vi "LDA_High_Convert_New.vi"(1 "Analysis Info cluster":T2[](array[typedef]) {"Sync Delay Time (s)" format="%.4f"; "Total Meas Time (s)" format="%_5g"; "Sd Error in Variance" format="%_3g"; "Skew_u" format="%_3g"; "% u'/U" format="%_3g"; "Sd Error in Mean" format="%_3g"; "Kurt_u" format="%_3g"; "u^4" format="%_3g"; "u^3" format="%_3g"; "U" format="%_3g"; "u^2" format="%_3g"}, 3 "Create Sync Index":bool, 4 "Time Trace in":T1[](array[typedef])) -> (5 "Analysis Info cluster Out":T2[](array[typedef]) {"Sync Delay Time (s)" format="%.4f"; "Total Meas Time (s)" format="%_5g"; "Sd Error in Variance" format="%_3g"; "Skew_u" format="%_3g"; "% u'/U" format="%_3g"; "Sd Error in Mean" format="%_3g"; "Kurt_u" format="%_3g"; "u^4" format="%_3g"; "u^3" format="%_3g"; "U" format="%_3g"; "u^2" format="%_3g"}, 6 "Error String":string, 7 "Diagnostic info":string[][](table), 8 "Time Trace out":T1[](array[typedef]), 9 "Sync Index":i32[](array[numeric]))   [LabVIEW 2021]
uses:
  Globals/LDA_meas_global_1.vi
  Globals/Meas_global.vi
  Globals/Preference_global.vi
  Globals/Plug_in_data_global.vi
  BSA_Type.ctl
  Globals/LDA_global.vi
  Controls/Inst_type.ctl
  Controls/Instrument_Array.ctl
  Controls/Analysis_info_cluster.ctl
  Controls/Time_Trace_Cluster.ctl
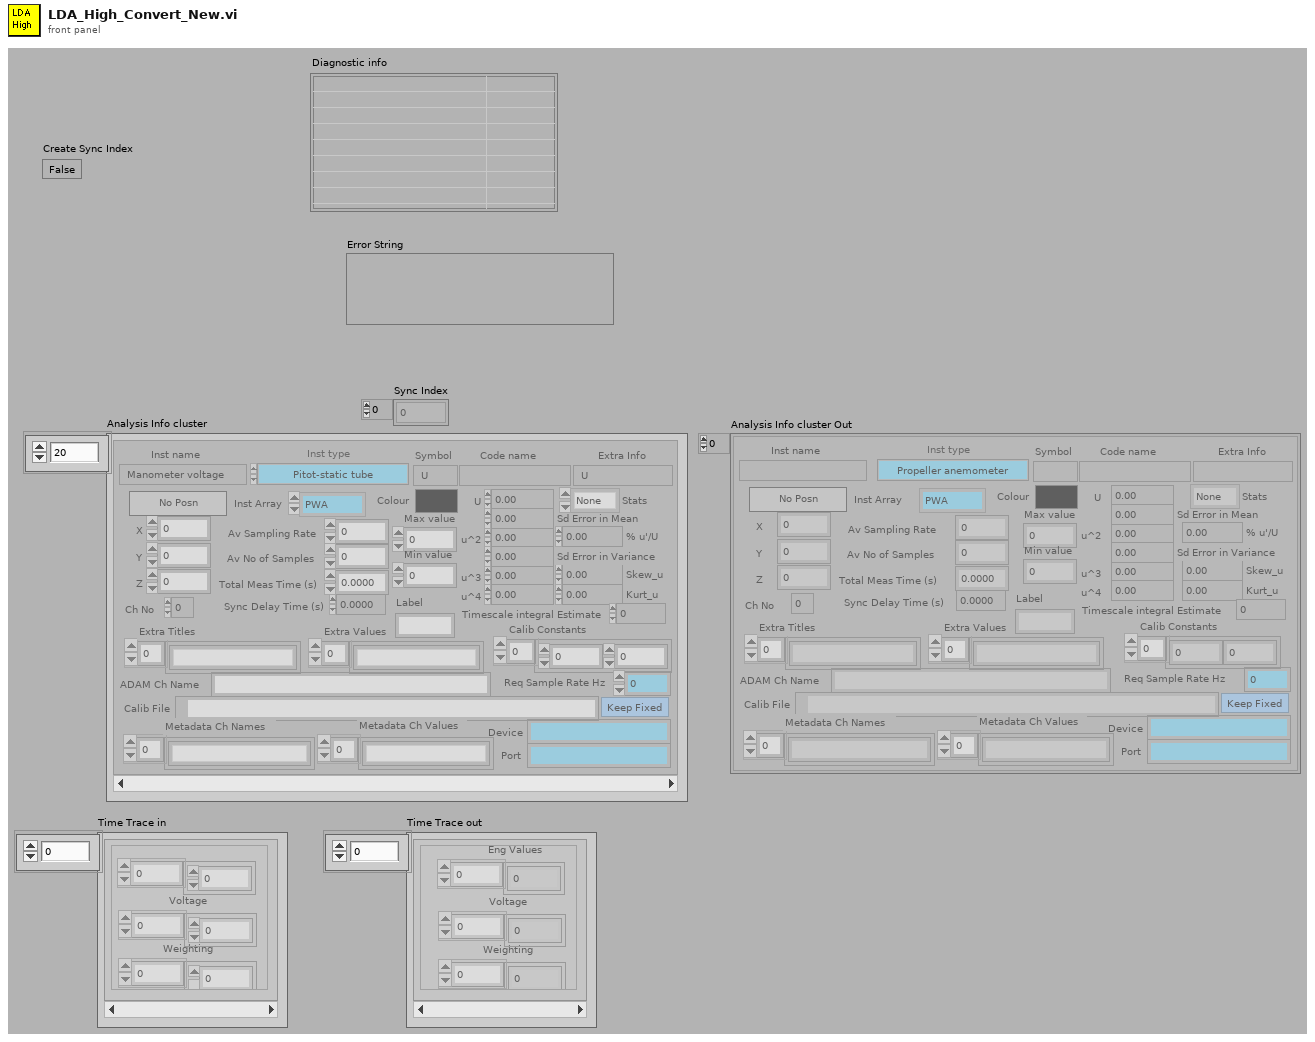
[diagram p1: front panel]
types:
  T1 = typedef "Time_Trace_Cluster.ctl" = cluster{"Weighting":dbl[], "Voltage":dbl[], "Eng Values":dbl[]}
  T2 = typedef "Analysis_info_cluster.ctl" = cluster{"Colour":u32, "Inst type":T3, "Inst name":string, "Symbol":string, "Code name":string, "Extra Info":string, "Inst Array":T4, "Extra Titles":string[], "Extra Values":string[], "U":dbl, "u^2":dbl, "u^3":dbl, "u^4":dbl, "Skew_u":dbl, "Kurt_u":dbl, "Sd Error in Mean":dbl, "% u'/U":dbl, "X":dbl, "Y":dbl, "Z":dbl, "Timescale integral Estimate":dbl, "Sd Error in Variance":dbl, "Calib File":path, "Calib Constants":dbl[], "Output Position":bool, "Stats":enum16{"None", "Basic", "Full"}, "Av Sampling Rate":dbl, "Av No of Samples":dbl, "Total Meas Time (s)":dbl, "ADAM Ch Name":string, "Max value":dbl, "Min value":dbl, "Req Sample Rate Hz":dbl, "Sync Delay Time (s)":dbl, "Ch No":i16, "Device":string, "Use Latest Calib":bool, "Port":string, "Metadata Ch Names":string[], "Metadata Ch Values":string[], "Label":string}
  T3 = typedef "Inst_type.ctl" = enum16{"Raw voltage", "Raw with zero offsetting", "Propeller anemometer", "Pressure Transducer", "Pitot-static tube", "Hot wire", "Cross wire 1", "Cross wire 2", "Generic Linear", "Generic Polynomial", "Generic BackPoly", "Fast FID", "Thermocouple", "Cold wire", "Pulsed Wire", "LDA Vel", "LDA Tran time", "LDA Arr time", "Microphone"}
  T4 = typedef "Instrument_Array.ctl" = enum16{"PWA", "LDA", "Analogue"}
  T5 = enum16{"Velocity", "Transit time", "Arrival time"}
  T6 = typedef "BSA_Type.ctl" = enum16{"57N11", "BSA F60"}
  T7 = typedef "LDA_Channel.ctl" = cluster{"Wavelength (nm)":dbl, "Vel Comp":string, "Max Velocity":dbl, "Min Velocity":dbl, "Max Record length":u16, "Signal gain (dB)":i16, "High voltage":i16, "Optics Conversion Factor":dbl, "Min Record length":u16, "Multiply Velocity by -1":bool, "Signal to Noise Ratio":string, "Validation Ratio":string, "Probe":string, "Laser":string, "BSA":string, "Lense":string, "Beam Separation (mm)":dbl, "Focal Length (mm)":dbl, "COLOUR":u32, "BSA IP":string, "Velocity Range (m/s)":dbl, "Centre Velocity (m/s)":dbl, "Unshifted mW":dbl, "Shifted mW":dbl, "Bandwidth Hz":dbl, "Req Sampling Rate Hz":dbl, "Ch":i32, "CenterFreq Hz":dbl, "Laser IP":string, "Sync Delay (s)":dbl}
  T8 = enum16{"Velocity", "Transit time", "Arrival time"}[]
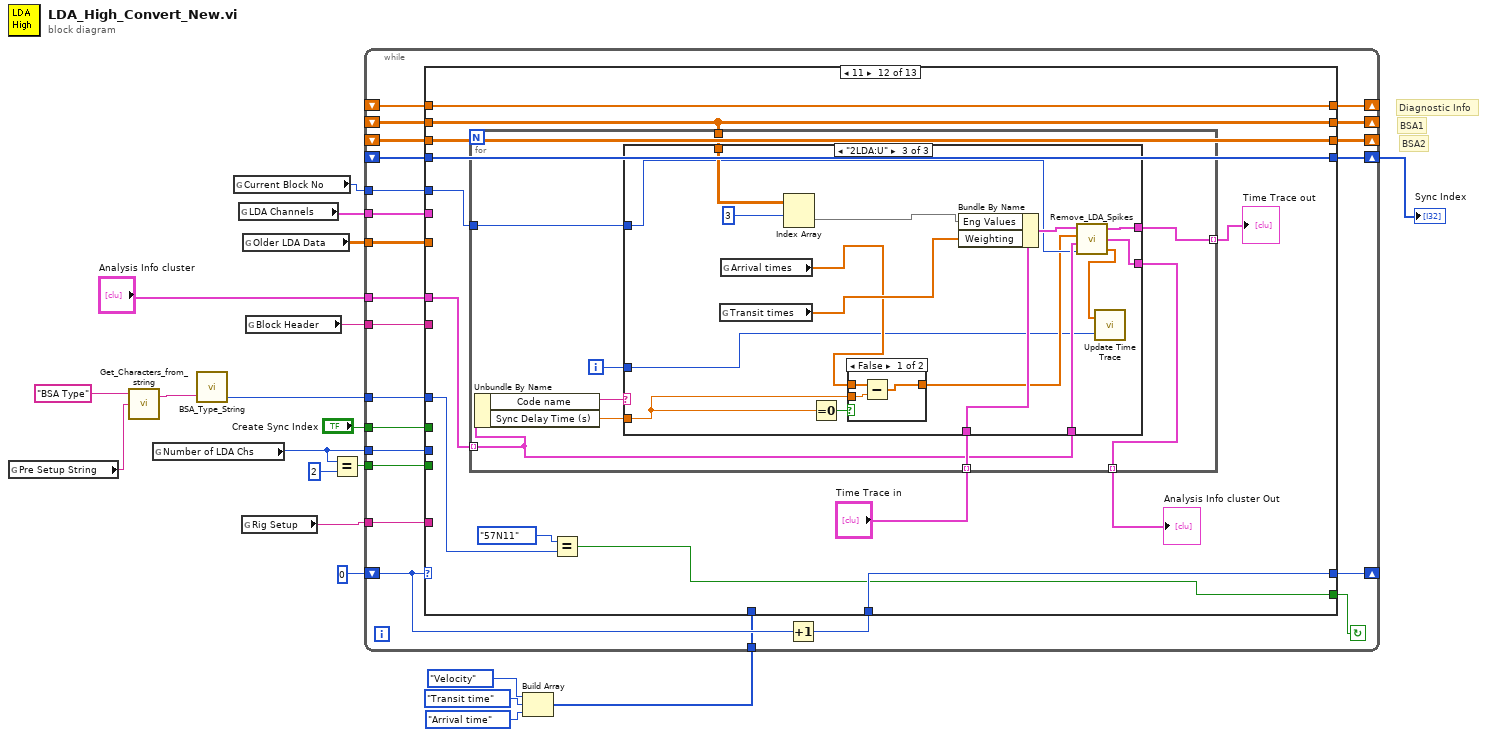
[diagram p0: block diagram]
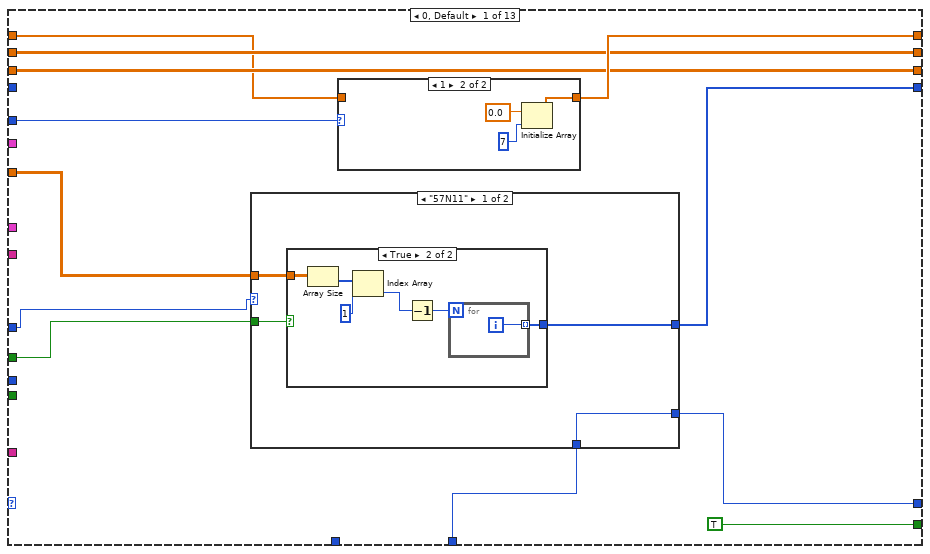
[diagram p2: hidden frame]
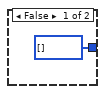
[diagram p4: hidden frame]
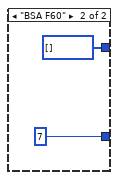
[diagram p5: hidden frame]
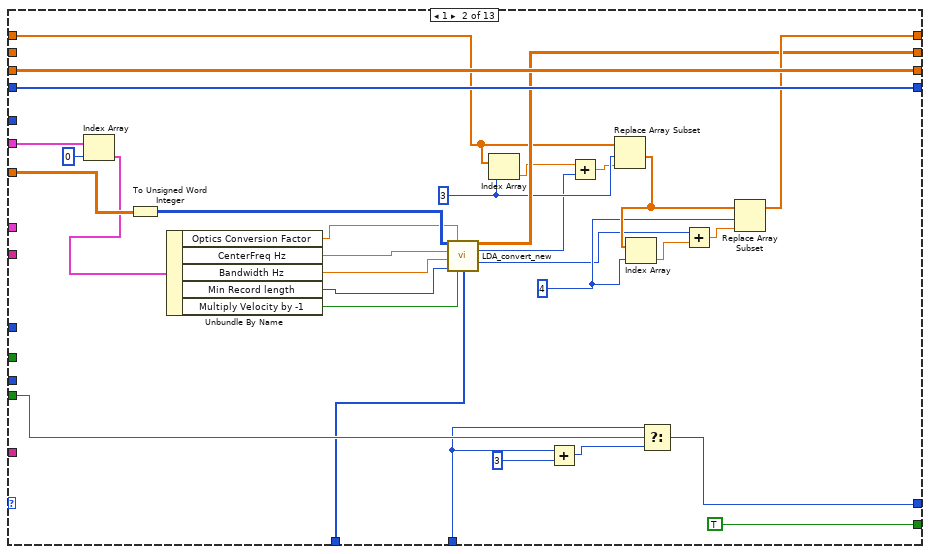
[diagram p6: hidden frame]
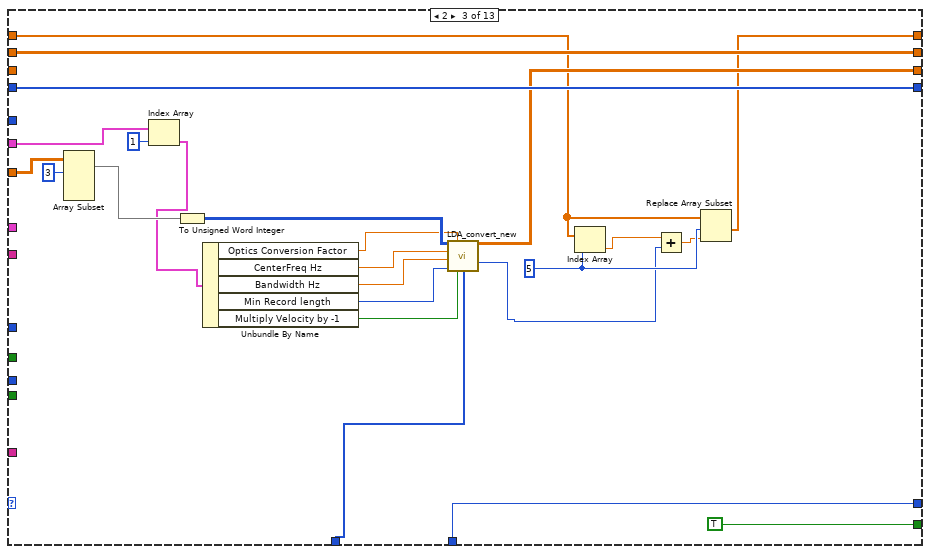
[diagram p7: hidden frame]
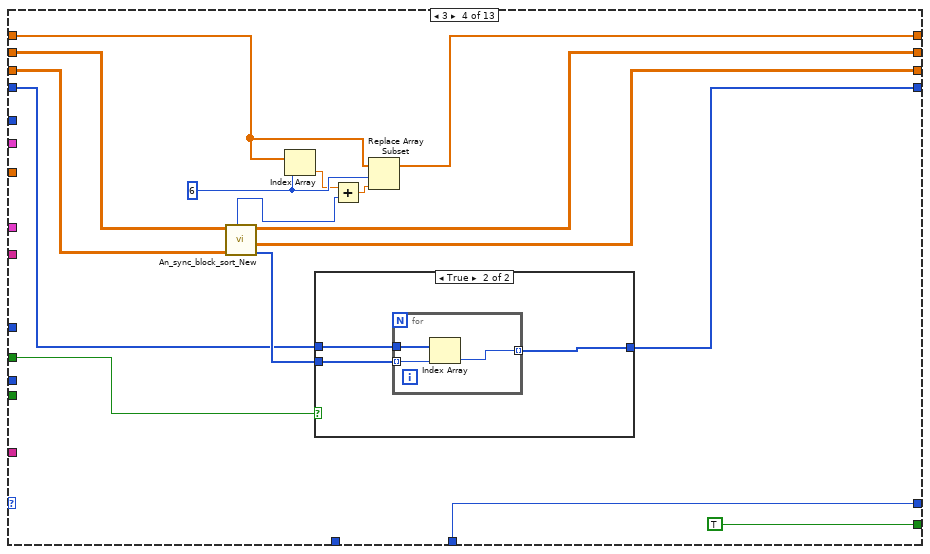
[diagram p8: hidden frame]
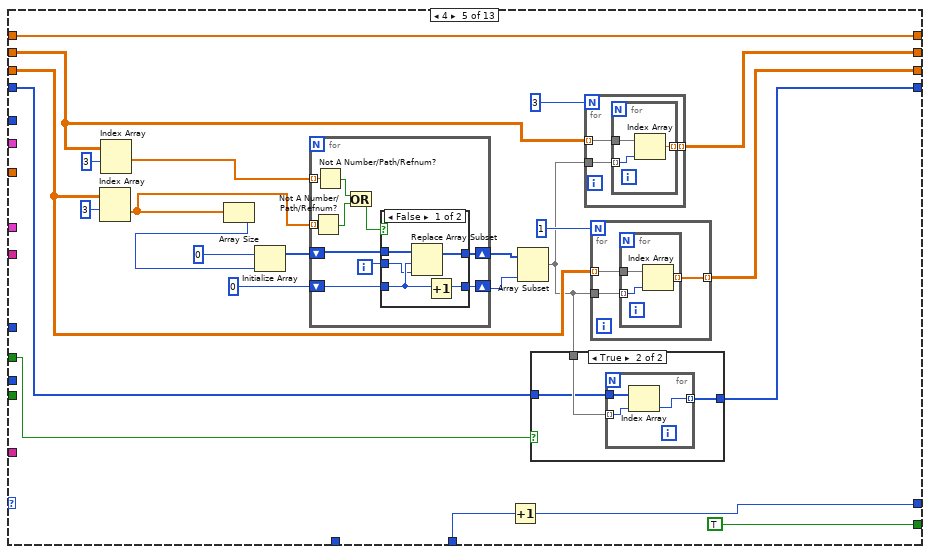
[diagram p10: hidden frame]
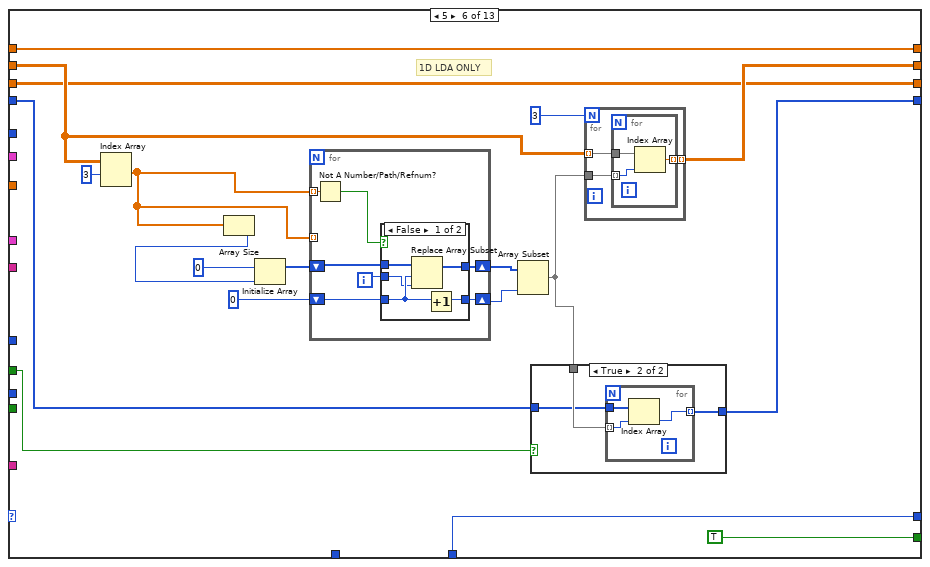
[diagram p13: hidden frame]
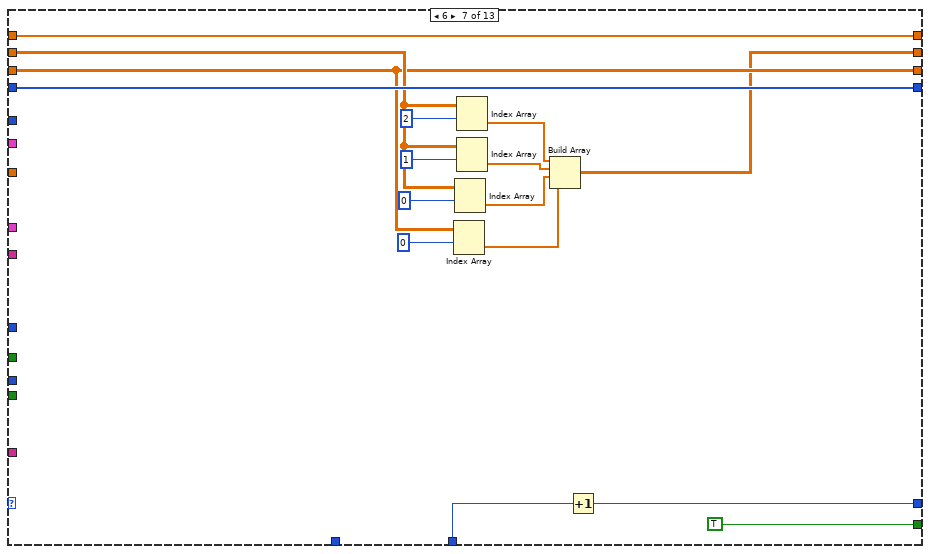
[diagram p16: hidden frame]
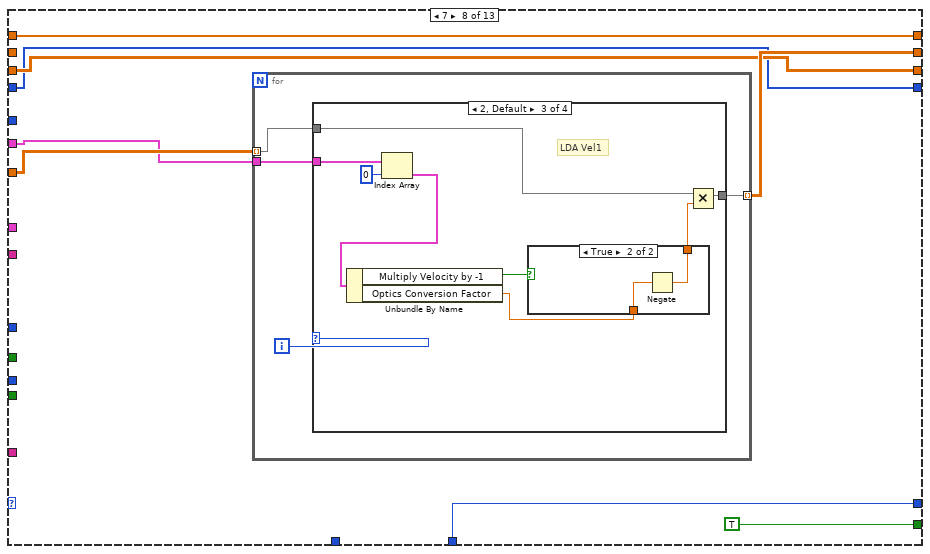
[diagram p17: hidden frame]
diagram:
  # "BSA2"
  # "BSA1"
  # "Diagnostic Info"
  n1 = global read "Meas_global.vi" "Pre Setup String"() -> (w7:string)
  n2 = call "Get_Characters_from_string.vi"("Input string"=w7, "Variable name"="BSA Type" ("Label for characters")) -> ("Value"=w5:string)  [unwired: 1 in, 1 out]
  n3 = global read "LDA_global.vi" "Number of LDA Chs"() -> (w3:i32)
  n4 = call "BSA_Type_String.vi"("BSA String in"=w5) -> ("BSA Type Out"=w4:T6)  [unwired: 1 in, 1 out]
  n5 = global read "Meas_global.vi" "Current Block No"() -> (w15:i32)
  n6 = global read "LDA_global.vi" "LDA Channels"() -> (w12:T7[])
  n7 = global read "Preference_global.vi" "Rig Setup"() -> (w14:string)
  n8 = global read "LDA_global.vi" "Older LDA Data"() -> (w13:dbl[][])
  n9 = global read "Plug_in_data_global.vi" "Block Header"() -> (w16:string)
  n10 = Equal?(x=w3, y=2) -> (x = y?=w18:bool)
  n11 = Build Array(T5."Velocity", T5."Transit time", T5."Arrival time") -> (w8:T8)
  n12 = while {
    tunnel: w3 -> [w30]
    tunnel: w18 -> [w31]
    tunnel: "Create Sync Index" -> [w38]
    shift-left: _ -> [w32]
    shift-right: [w39] -> w17
    shift-left: _ -> [w35]
    shift-right: [w34] -> _
    shift-left: _ -> [w37]
    shift-right: [w36] -> _
    shift-left: _ -> [w33]
    shift-right: [w40] -> _
    shift-left: 0 -> [w42]
    shift-right: [w29] -> _
    tunnel: w16 -> [w28]
    tunnel: w15 -> [w27]
    tunnel: w14 -> [w26]
    tunnel: w13 -> [w25]
    tunnel: w12 -> [w24]
    tunnel: w8 -> [w23]
    tunnel: w4 -> [w22]
    tunnel: "Analysis Info cluster" -> [w21]
    stop <- w43 continue-if-true
    n13 = Increment(x=w42) -> (x+1=w41:i32)
    n14 = case shown="11" w42 {
      tunnel: [TRUE TRUE TRUE TRUE TRUE TRUE TRUE TRUE TRUE TRUE w365 w420 FALSE] -> w43
      tunnel: w41 -> [w48 w97 w124 w143 w153 w229 w272 w277 w328 w337 w364 w429 w492]
      tunnel: [w54 w101 w119 w138 w154 w214 w258 w278 w319 w336 w373 w426 w491] -> w40
      tunnel: [w53 w102 w127 w134 w159 w216 w271 w279 w330 w338 w366 w427 w494] -> w39
      tunnel: w38 -> [w52 _ _ w137 w161 w218 _ _ _ _ _ _ _]
      tunnel: w37 -> [w51 _ w126 w142 w163 w220 w263 _ w314 w335 w371 w423 w485]
      tunnel: [w51 w100 w126 w140 w162 w219 w261 w281 w314 w334 w370 w423 w485] -> w36
      tunnel: w35 -> [w50 w103 _ w141 w158 w212 w262 w280 w329 w333 w368 w428 w493]
      tunnel: [w50 w103 w125 w139 w157 w212 w262 w280 w329 w333 w369 w428 w493] -> w34
      tunnel: w33 -> [w47 w94 w120 w132 w154 w214 w258 w278 w320 w336 w372 w426 w491]
      tunnel: w32 -> [_ w102 w127 w135 w160 w217 w271 w279 w330 w338 w367 w427 w494]
      tunnel: w31 -> [_ w99 _ _ _ _ _ _ _ _ w361 _ _]
      tunnel: w30 -> [_ _ _ _ _ _ _ _ _ _ w363 _ _]
      tunnel: [w49 w98 w124 w143 w152 w229 w260 w277 w328 w337 w360 w429 w492] -> w29
      tunnel: w28 -> [_ _ _ _ _ _ _ _ _ _ _ _ _]
      tunnel: w27 -> [w46 _ _ _ _ _ _ _ _ _ w362 w422 w487]
      tunnel: w26 -> [_ _ _ _ _ _ _ _ _ _ _ _ _]
      tunnel: w25 -> [w45 w83 w115 _ _ _ _ w275 _ _ _ _ _]
      tunnel: w24 -> [_ w82 w107 _ _ _ _ w274 _ _ _ _ _]
      tunnel: w23 -> [_ w74 w114 _ _ _ _ _ _ _ _ _ _]
      tunnel: w22 -> [w44 _ _ _ _ _ _ _ _ w332 w359 w421 _]
      tunnel: w21 -> [_ _ _ _ _ _ _ _ _ _ _ w419 w481]
      frame 0, Default {
        n15 = case shown="\"57N11\"" w44 {
          tunnel: [w63 i32[] []] -> w53
          tunnel: w52 -> [w62 _]
          tunnel: w45 -> [w61 _]
          tunnel: [w60 7] -> w49
          tunnel: w48 -> [w60 _]
          frame "57N11" {
            n16 = case shown="True" w62 {
              tunnel: [i32[] [] w70] -> w63
              tunnel: w61 -> [_ w69]
              frame False {
              }
              frame True {
                n17 = Array Size(array=w69) -> (size(s)=w68:i32[])
                n18 = Index Array(array=w68, index=1 ("Index")) -> (element=w67:i32)
                n19 = Decrement(x=w67) -> (x-1=w66:i32)
                n20 = for {
                  N: w66 -> [_]
                  tunnel: [w71] -> w70 mode=indexing
                  i -> [w71]
                }
              }
            }
          }
          frame "BSA F60" {
          }
        }
        n21 = case shown="1" w46 {
          tunnel: [w56 w57] -> w54
          tunnel: w47 -> [w56 _]
          frame 2, Default {
          }
          frame 1 {
            n22 = Initialize Array(0.0, 7 ("Dimension Size")) -> (w57:dbl[])
          }
        }
      }
      frame 1 {
        w88 = 4 ("Index")
        w93 = 3 ("Index")
        n23 = Index Array(array=w82, index=0) -> (element=w80:T7)
        n24 = To Unsigned Word Integer(number=w83) -> (unsigned 16bit integer=w84:u16[][])
        n25 = Unbundle By Name(w80) -> ("Optics Conversion Factor"=w79:dbl, "CenterFreq Hz"=w78:dbl, "Bandwidth Hz"=w77:dbl, "Min Record length"=w76:u16, "Multiply Velocity by -1"=w75:bool)
        n26 = call "LDA_convert_new.vi"("binary data"=w84, "Calibration factor"=w79, "Centre frequency"=w78, "Bandwidth"=w77, "Record length (RL)"=w76, "Multiply Velocity by -1"=w75, "data type"=w74) -> ("Converted results"=w100:dbl[][], "No of cntr resets"=w91:i32, "No invalid"=w86:i32)  [unwired: 1 in, 5 out]
        n27 = Index Array(array=w94, index=w93) -> (element=w92:dbl)
        n28 = Add(x=w97, y=3) -> (x+y=w95:i32)
        n29 = Add(x=w92, y=w91) -> (x+y=w90:dbl)
        n30 = Replace Array Subset(array=w94, new element=w90, index=w93) -> (w89:dbl[])
        n31 = Index Array(array=w89, index=w88) -> (element=w85:dbl)
        n32 = Select(t=w97, s=w99, f=w95) -> (s? t:f=w98:i32)
        n33 = Add(x=w86, y=w85) -> (x+y=w87:dbl)
        n34 = Replace Array Subset(array=w89, new element=w87, index=w88) -> (w101:dbl[])
      }
      frame 2 {
        w123 = 5 ("Index")
        n35 = Array Subset(array=w115, index (row)=3 ("index")) -> (w117:dbl[][])  [unwired: 3 in]
        n36 = Index Array(array=w107, index=1) -> (element=w106:T7)
        n37 = To Unsigned Word Integer(number=w117) -> (unsigned 16bit integer=w116:u16[][])
        n38 = Unbundle By Name(w106) -> ("Optics Conversion Factor"=w113:dbl, "CenterFreq Hz"=w112:dbl, "Bandwidth Hz"=w111:dbl, "Min Record length"=w110:u16, "Multiply Velocity by -1"=w109:bool)
        n39 = call "LDA_convert_new.vi"("binary data"=w116, "Calibration factor"=w113, "Centre frequency"=w112, "Bandwidth"=w111, "Record length (RL)"=w110, "Multiply Velocity by -1"=w109, "data type"=w114) -> ("Converted results"=w125:dbl[][], "No invalid"=w118:i32)  [unwired: 1 in, 6 out]
        n40 = Index Array(array=w120, index=w123) -> (element=w122:dbl)
        n41 = Add(x=w122, y=w118) -> (x+y=w121:dbl)
        n42 = Replace Array Subset(array=w120, new element=w121, index=w123) -> (w119:dbl[])
      }
      frame 3 {
        w133 = 6 ("Index")
        n43 = call "An_sync_block_sort_New.vi"("BSA 2"=w141, "BSA 1"=w142) -> ("Analogue Sync Index"=w136:i32[], "BSA 2 Sync"=w139:dbl[][], "BSA 1 Sync"=w140:dbl[][], "No of slips"=w129:i32)  [unwired: 4 out]
        n44 = Index Array(array=w132, index=w133) -> (element=w130:dbl)
        n45 = case shown="True" w137 {
          tunnel: w136 -> [_ w148]
          tunnel: w135 -> [w145 w147]
          tunnel: [w145 w146] -> w134
          frame False {
          }
          frame True {
            n46 = for {
              tunnel: w148 -> [w151] mode=indexing
              tunnel: w147 -> [w150]
              tunnel: [w149] -> w146 mode=indexing
              n47 = Index Array(array=w150, index=w151) -> (element=w149:i32)
            }
          }
        }
        n48 = Add(x=w130, y=w129) -> (x+y=w131:dbl)
        n49 = Replace Array Subset(array=w132, new element=w131, index=w133) -> (w138:dbl[])
      }
      frame 4 {
        n50 = Index Array(array=w158, index (row)=3 ("Index")) -> (element=w166:dbl[])  [unwired: 1 in]
        n51 = Index Array(array=w163, index (row)=3 ("Index")) -> (element=w165:dbl[])  [unwired: 1 in]
        n52 = Array Size(array=w166) -> (size(s)=w168:i32)
        n53 = Initialize Array(0, w168) -> (w170:i32[])
        n54 = for {
          shift-right: [w203] -> w172
          shift-left: w170 -> [w204]
          shift-right: [w201] -> w167
          shift-left: 0 -> [w202]
          tunnel: w166 -> [w197] mode=indexing
          tunnel: w165 -> [w196] mode=indexing
          i -> [w200]
          n55 = Not A Number/Path/Refnum?(number/path/refnum=w197) -> (NaN/Path/Refnum?=w199:bool)
          n56 = Not A Number/Path/Refnum?(number/path/refnum=w196) -> (NaN/Path/Refnum?=w198:bool)
          n57 = Or(x=w198, y=w199) -> (x .or. y?=w195:bool)
          n58 = case shown="False" w195 {
            tunnel: w204 -> [w209 w211]
            tunnel: [w208 w211] -> w203
            tunnel: w202 -> [w207 w210]
            tunnel: [w206 w210] -> w201
            tunnel: w200 -> [w205 _]
            frame False {
              n59 = Replace Array Subset(array=w209, new element=w205, index=w207) -> (w208:i32[])
              n60 = Increment(x=w207) -> (x+1=w206:i32)
            }
            frame True {
            }
          }
        }
        n61 = Increment(x=w153) -> (x+1=w152:i32)
        n62 = Array Subset(array=w172, length=w167) -> (w155:i32[])  [unwired: 1 in]
        n63 = case shown="True" w161 {
          tunnel: w155 -> [_ w185]
          tunnel: w160 -> [w182 w184]
          tunnel: [w182 w183] -> w159
          frame False {
          }
          frame True {
            n64 = for {
              tunnel: w185 -> [w187] mode=indexing
              tunnel: w184 -> [w188]
              tunnel: [w186] -> w183 mode=indexing
              n65 = Index Array(array=w188, index=w187) -> (element=w186:i32)
            }
          }
        }
        n66 = for {
          N: 3 -> [_]
          tunnel: w163 -> [w191] mode=indexing
          tunnel: w155 -> [w190]
          tunnel: [w189] -> w162 mode=indexing
          n67 = for {
            tunnel: w190 -> [w193] mode=indexing
            tunnel: w191 -> [w194]
            tunnel: [w192] -> w189 mode=indexing
            n68 = Index Array(array=w194, index=w193) -> (element=w192:dbl)
          }
        }
        n69 = for {
          N: 1 -> [_]
          tunnel: w155 -> [w178]
          tunnel: w158 -> [w177] mode=indexing
          tunnel: [w176] -> w157 mode=indexing
          n70 = for {
            tunnel: w178 -> [w180] mode=indexing
            tunnel: w177 -> [w181]
            tunnel: [w179] -> w176 mode=indexing
            n71 = Index Array(array=w181, index=w180) -> (element=w179:dbl)
          }
        }
      }
      frame 5 {
        # "1D LDA ONLY"
        n72 = Index Array(array=w220, index (row)=3 ("Index")) -> (element=w213:dbl[])  [unwired: 1 in]
        n73 = Array Size(array=w213) -> (size(s)=w223:i32)
        n74 = Initialize Array(0, w223) -> (w225:i32[])
        n75 = for {
          shift-right: [w249] -> w227
          shift-left: w225 -> [w250]
          shift-right: [w247] -> w222
          shift-left: 0 -> [w248]
          tunnel: w213 -> [_] mode=indexing
          tunnel: w213 -> [w245] mode=indexing
          i -> [w246]
          n76 = Not A Number/Path/Refnum?(number/path/refnum=w245) -> (NaN/Path/Refnum?=w244:bool)
          n77 = case shown="False" w244 {
            tunnel: w250 -> [w255 w257]
            tunnel: [w254 w257] -> w249
            tunnel: w248 -> [w253 w256]
            tunnel: [w252 w256] -> w247
            tunnel: w246 -> [w251 _]
            frame False {
              n78 = Replace Array Subset(array=w255, new element=w251, index=w253) -> (w254:i32[])
              n79 = Increment(x=w253) -> (x+1=w252:i32)
            }
            frame True {
            }
          }
        }
        n80 = Array Subset(array=w227, length=w222) -> (w215:i32[])  [unwired: 1 in]
        n81 = case shown="True" w218 {
          tunnel: w215 -> [_ w234]
          tunnel: w217 -> [w231 w233]
          tunnel: [w231 w232] -> w216
          frame False {
          }
          frame True {
            n82 = for {
              tunnel: w234 -> [w236] mode=indexing
              tunnel: w233 -> [w237]
              tunnel: [w235] -> w232 mode=indexing
              n83 = Index Array(array=w237, index=w236) -> (element=w235:i32)
            }
          }
        }
        n84 = for {
          N: 3 -> [_]
          tunnel: w220 -> [w240] mode=indexing
          tunnel: w215 -> [w239]
          tunnel: [w238] -> w219 mode=indexing
          n85 = for {
            tunnel: w239 -> [w242] mode=indexing
            tunnel: w240 -> [w243]
            tunnel: [w241] -> w238 mode=indexing
            n86 = Index Array(array=w243, index=w242) -> (element=w241:dbl)
          }
        }
      }
      frame 6 {
        n87 = Index Array(array=w262, index (row)=0) -> (element=w259:dbl[])  [unwired: 1 in]
        n88 = Index Array(array=w263, index (row)=0) -> (element=w264:dbl[])  [unwired: 1 in]
        n89 = Index Array(array=w263, index (row)=2) -> (element=w266:dbl[])  [unwired: 1 in]
        n90 = Index Array(array=w263, index (row)=1) -> (element=w265:dbl[])  [unwired: 1 in]
        n91 = Build Array(w266, w265, w264, w259) -> (w261:dbl[][])
        n92 = Increment(x=w272) -> (x+1=w260:i32)
      }
      frame 7 {
        n93 = for {
          tunnel: [w284] -> w281 mode=indexing
          tunnel: w275 -> [w283] mode=indexing
          tunnel: w274 -> [w282]
          i -> [w285]
          n94 = case shown="2, Default" w285 {
            tunnel: w283 -> [w286 w287 w295 w306]
            tunnel: [w286 w287 w294 w305] -> w284
            tunnel: w282 -> [_ _ w292 w301]
            frame 0 {
              # "Arrival Times"
            }
            frame 1 {
              # "Transit Times"
            }
            frame 2, Default {
              # "LDA Vel1"
              n95 = Index Array(array=w292, index=0) -> (element=w291:T7)
              n96 = Unbundle By Name(w291) -> ("Multiply Velocity by -1"=w290:bool, "Optics Conversion Factor"=w289:dbl)
              n97 = case shown="True" w290 {
                tunnel: w289 -> [w296 w298]
                tunnel: [w296 w297] -> w293
                frame False {
                }
                frame True {
                  n98 = Negate(x=w298) -> (-x=w297:dbl)
                }
              }
              n99 = Multiply(x=w295, y=w293) -> (x*y=w294:dbl[])
            }
            frame 3 {
              # "LDA Vel2"
              n100 = Index Array(array=w301, index=1) -> (element=w303:T7)
              n101 = Unbundle By Name(w303) -> ("Multiply Velocity by -1"=w300:bool, "Optics Conversion Factor"=w299:dbl)
              n102 = case shown="True" w300 {
                tunnel: w299 -> [w307 w309]
                tunnel: [w307 w308] -> w304
                frame False {
                }
                frame True {
                  n103 = Negate(x=w309) -> (-x=w308:dbl)
                }
              }
              n104 = Multiply(x=w306, y=w304) -> (x*y=w305:dbl[])
            }
          }
        }
      }
      frame 8 {
        w323 = 1 ("Index")
        w325 = 0 ("Index")
        n105 = Index Array(array=w314, index (row)=0 ("Index")) -> (element=w311:dbl[])  [unwired: 1 in]
        n106 = Array Size(array=w311) -> (size(s)=w312:i32)
        n107 = Decrement(x=w312) -> (x-1=w313:i32)
        n108 = Array Size(array=w314) -> (size(s)=w327:i32[])
        n109 = Index Array(array=w311, index=w313) -> (element=w310:dbl)
        n110 = Index Array(array=w320, index=w325) -> (element=w324:dbl)
        n111 = Index Array(array=w327, index=1 ("Index")) -> (element=w318:i32)
        n112 = Add(x=w324, y=w310) -> (x+y=w316:dbl)
        n113 = Replace Array Subset(array=w320, new element=w316, index=w325) -> (w321:dbl[])
        n114 = Index Array(array=w321, index=w323) -> (element=w322:dbl)
        n115 = Add(x=w322, y=w318) -> (x+y=w317:dbl)
        n116 = Replace Array Subset(array=w321, new element=w317, index=w323) -> (w319:dbl[])
      }
      frame 9 {
        n117 = for {
          tunnel: w335 -> [w342] mode=indexing
          tunnel: [w341] -> w334 mode=indexing
          tunnel: w332 -> [w340]
          i -> [w343]
          n118 = case shown="2, Default" w343 {
            tunnel: w342 -> [w345 w351 w358]
            tunnel: [w345 w352 w358] -> w341
            tunnel: w340 -> [w346 w353 _]
            frame 0 {
              n119 = case shown="\"57N11\"" w346 {
                tunnel: [w347 w350] -> w344
                tunnel: w345 -> [w349 w350]
                frame "57N11" {
                  n120 = Multiply(x=0.001, y=w349) -> (x*y=w347:dbl[])
                }
                frame "BSA F60" {
                }
              }
              n121 = global write "LDA_meas_global_1.vi" "Arrival times"(w344) -> ()
            }
            frame 1 {
              # "Transit Times"
              n122 = case shown="\"BSA F60\"" w353 {
                tunnel: [w354 w355] -> w352
                tunnel: w351 -> [w354 w357]
                frame "57N11" {
                }
                frame "BSA F60" {
                  n123 = Multiply(x=1000000.0, y=w357) -> (x*y=w355:dbl[])
                }
              }
              n124 = global write "LDA_meas_global_1.vi" "Transit times"(w352) -> ()
            }
            frame 2, Default {
              # "LDA Vel2"
              # "LDA Vel1"
            }
          }
        }
      }
      frame 10 {
        n125 = stacked-sequence {
          seq-local: [w378 _ _] -> [_ _ w413]
          seq-local: [w379 _ _] -> [_ _ w412]
          seq-local: [w377 _ _] -> [_ w411 _]
          tunnel: [w376 _ _] -> w373
          tunnel: w372 -> [w376 _ _]
          tunnel: w371 -> [_ _ w416]
          tunnel: [_ _ w416] -> w370
          tunnel: [_ _ w415] -> w369
          tunnel: w368 -> [_ _ w415]
          tunnel: w367 -> [_ _ w414]
          tunnel: [_ _ w414] -> w366
          tunnel: [TRUE _ _] -> w365
          tunnel: w364 -> [w385 _ _]
          tunnel: [w385 _ _] -> w360
          tunnel: w359 -> [w390 _ _]
          tunnel: w363 -> [w382 _ _]
          tunnel: w362 -> [w384 _ _]
          tunnel: w361 -> [_ _ _]
          frame #0 {
            n126 = Divide(x=w376, y=w384) -> (x/y=w374:dbl[])
            n127 = case shown="\"BSA F60\"" w390 {
              tunnel: w382 -> [w401 _]
              tunnel: "No of:Resets::" -> [w400 _]
              tunnel: "No of:Invalid:Bursts BSA 1:" -> [w399 _]
              tunnel: "No of:invalid:Bursts BSA 2:" -> [w398 _]
              tunnel: "No of:Slips:in Arrival:times" -> [w397 _]
              tunnel: w384 -> [w396 _]
              tunnel: [w395 string[] []] -> w379
              frame "57N11" {
                n128 = case shown="1, Default" w401 {
                  tunnel: w400 -> [w406 w409]
                  tunnel: w399 -> [w405 w408]
                  tunnel: w398 -> [w404 _]
                  tunnel: w397 -> [w403 _]
                  tunnel: w396 -> [_ _]
                  tunnel: [w402 w407] -> w395
                  frame 2 {
                    n129 = Build Array(w406, w405, w404, w403) -> (w402:string[])
                  }
                  frame 1, Default {
                    n130 = Build Array(w409, w408) -> (w407:string[])
                  }
                }
              }
              frame "BSA F60" {
              }
            }
            n131 = Array Size(array=w379) -> (size(s)=w383:i32)
            n132 = Array Subset(array=w374, index=3, length=w383) -> (w381:dbl[])
            n133 = Number To Fractional String(number=w381, precision (6)=i16 2) -> (F-format string=w378:string[])  [unwired: 2 out]
            n134 = for {
              tunnel: w379 -> [w394] mode=indexing
              tunnel: w378 -> [w393] mode=indexing
              tunnel: [w392] -> w377 mode=indexing
              n135 = Build Array(w394, w393) -> (w392:string[])
            }
          }
          frame #1 {
            n136 = global write "Meas_global.vi" "Diagnostic info"(w411) -> ()
            "Diagnostic info" <- w411
          }
          frame #2 {
            n137 = global write "LDA_meas_global_1.vi" "LDA Results file Values"(w413) -> ()
            n138 = global write "LDA_meas_global_1.vi" "LDA Results file headers"(w412) -> ()
          }
        }
      }
      frame 11 {
        n139 = for {
          tunnel: [w437] -> w424 mode=indexing
          tunnel: w423 -> [w436]
          tunnel: "Time Trace in" -> [w435] mode=indexing
          tunnel: [w434] -> w418 mode=indexing
          tunnel: w422 -> [w433]
          tunnel: w419 -> [w431] mode=indexing
          i -> [w430]
          n140 = Unbundle By Name(w431) -> ("Code name"=w438:string, "Sync Delay Time (s)"=w432:dbl)
          n141 = case shown="\"2LDA:U\"" w438 {
            tunnel: [w440 w449 w469] -> w437
            tunnel: w431 -> [w440 w447 w470]
            tunnel: w436 -> [_ w455 w476]
            tunnel: w435 -> [w439 w452 w475]
            tunnel: [w439 w450 w471] -> w434
            tunnel: w433 -> [_ w448 w468]
            tunnel: w432 -> [_ w445 w466]
            tunnel: w430 -> [_ w441 w461]
            frame "False", Default {
            }
            frame "1LDA:U" {
              n142 = global read "LDA_meas_global_1.vi" "Arrival times"() -> (w444:dbl[])
              n143 = global read "LDA_meas_global_1.vi" "Transit times"() -> (w456:dbl[])
              n144 = Index Array(array=w455, index (row)=2) -> (element=w453:dbl[])  [unwired: 1 in]
              n145 = Equal To 0?(x=w445) -> (x = 0?=w446:bool)
              n146 = case shown="False" w446 {
                tunnel: [w458 w460] -> w443
                tunnel: w444 -> [w459 w460]
                tunnel: w445 -> [w457 _]
                frame False {
                  n147 = Subtract(x=w459, y=w457) -> (x-y=w458:dbl[])
                }
                frame True {
                }
              }
              n148 = Bundle By Name(cluster=w452, "Eng Values"=w453, "Weighting"=w456) -> (w451:T1)
              n149 = call "Remove_LDA_Spikes.vi"("Current Block Number"=w448, "Analaysis info Cluster"=w447, "Time (s) In"=w443, "Time Trace In"=w451) -> ("Time (s) Out"=w442:dbl[], "Analaysis info Cluster Out"=w449:T2, "Time trace Out"=w450:T1)
              n150 = call "Update Time Trace.vi"("Channel Index"=w441, "Time (s)"=w442) -> ()  [unwired: 1 in]
            }
            frame "2LDA:U" {
              n151 = global read "LDA_meas_global_1.vi" "Transit times"() -> (w474:dbl[])
              n152 = global read "LDA_meas_global_1.vi" "Arrival times"() -> (w465:dbl[])
              n153 = Index Array(array=w476, index (row)=3) -> (element=w473:dbl[])  [unwired: 1 in]
              n154 = Equal To 0?(x=w466) -> (x = 0?=w467:bool)
              n155 = case shown="False" w467 {
                tunnel: [w478 w480] -> w463
                tunnel: w465 -> [w479 w480]
                tunnel: w466 -> [w477 _]
                frame False {
                  n156 = Subtract(x=w479, y=w477) -> (x-y=w478:dbl[])
                }
                frame True {
                }
              }
              n157 = Bundle By Name(cluster=w475, "Eng Values"=w473, "Weighting"=w474) -> (w472:T1)
              n158 = call "Remove_LDA_Spikes.vi"("Current Block Number"=w468, "Analaysis info Cluster"=w470, "Time (s) In"=w463, "Time Trace In"=w472) -> ("Time (s) Out"=w462:dbl[], "Analaysis info Cluster Out"=w469:T2, "Time trace Out"=w471:T1)
              n159 = call "Update Time Trace.vi"("Channel Index"=w461, "Time (s)"=w462) -> ()  [unwired: 1 in]
            }
          }
        }
        "Analysis Info cluster Out" <- w424
        "Time Trace out" <- w418
        n160 = Equal?(x=BSA_Type."57N11" ("BSA Type"), y=w421) -> (x = y?=w420:bool)
      }
      frame 12 {
        n161 = Array Size(array=w485) -> (size(s)=w484:i32[])
        n162 = Index Array(array=w484, index=1) -> (element=w482:i32)
        n163 = for {
          shift-right: [w503] -> w488
          shift-left: "" -> [w504]
          tunnel: 4 ("Index") -> [w510]
          tunnel: w491 -> [w507]
          tunnel: w482 -> [w502]
          tunnel: w481 -> [w500] mode=indexing
          tunnel: w487 -> [w495]
          i -> [w509]
          n164 = Unbundle By Name(w500) -> ("Inst name"=w499:string)
          n165 = Add(x=w510, y=w509) -> (x+y=w508:i32)
          n166 = Index Array(array=w507, index=w508) -> (element=w497:dbl)
          n167 = Divide(x=w497, y=w495) -> (x/y=w496:dbl)
          n168 = Divide(x=w496, y=w502) -> (x/y=w506:dbl)
          n169 = Greater?(x=w506, y=0.5) -> (0:w498:bool)
          n170 = case shown="True" w498 {
            tunnel: w504 -> [w511 w517]
            tunnel: [w511 w516] -> w503
            tunnel: w496 -> [_ w515]
            tunnel: w502 -> [_ w514]
            tunnel: "%s has an average of %.0f invalid bursts for a block size of %.0f.\n" ("Format String") -> [_ w513]
            tunnel: w499 -> [_ w512]
            frame False {
            }
            frame True {
              n171 = Format Into String(format string=w513, initial string=w517, w512, w515, w514) -> (resulting string=w516:string)  [unwired: 1 in, 1 out]
            }
          }
        }
        "Error String" <- w488
      }
    }
  }
  "Sync Index" <- w17
